vi "NI VeriStand - Send Workspace Tool Message.vi"   [LabVIEW 2020, in "NI_VS Project ExecutionAPI.lvlib"]
doc: "Sends a message or command to a Workspace tool for an NI VeriStand project, as well as data required by the case that handles the command. You can use this method with any Workspace tool that registers to receive the command you specify."
uses:
  <vilib>/NI VeriStand/Execution/Project/NI_VS Project ExecutionAPI.lvlib
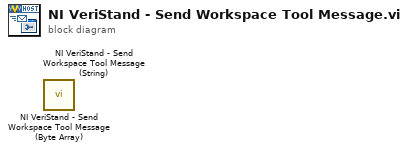
[diagram p0: block diagram]
diagram:
  n1 = call <vilib>:"NI VeriStand - Send Workspace Tool Message (Byte Array).vi"() -> ()  [unwired: 9 in, 3 out]
  n2 = call <vilib>:"NI VeriStand - Send Workspace Tool Message (String).vi"() -> ()  [unwired: 9 in, 3 out]
